vi "Fade.vi"(6 "Fade (Exponential)":T1, 8 "error in":errorcluster, 9 "Target Transparency (0)":u8, 10 "Fade time (ms)":variant, 11 "VI Reference (calling VI)":refnum<vi>) -> (0 "error out":errorcluster, 3 "dup VI Reference":refnum<vi>)   [LabVIEW 2012]
doc: "Produces a fade in or out, from the actual value to the target transparency. Use this generic VI when you start from an unknown transparency value.\n\nVariant (%) can be a numeric or a string containing a number. This allows the use of string-based arguments without the need to convert to a number."
uses:
  _fadetype.ctl
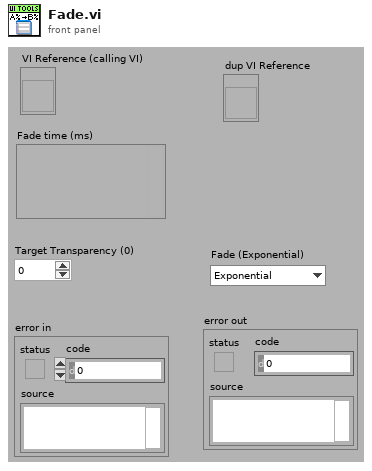
[diagram p1: front panel]
types:
  T1 = typedef "_fadetype.ctl" = enum16{"Exponential", "Linear"}
  T2 = typedef "Type Descriptor Enumeration__ogtk.ctl" = enum8{"<Null>", "I8", "I16", "I32", "I64", "U8", "U16", "U32", "U64", "SGL", "DBL", "EXT", "CSG", "CDB", "CXT", "0x0F", "0x10", "0x11", "0x12", "0x13", "0x14", "Enum U8", "Enum U16", "Enum U32", "Enum U64", "SGL PQ", "DBL PQ", "EXT PQ", "CSG PQ", "CDB PQ", "CXT PQ", "0x1F", "0x20", "Boolean", "0x22", "0x23", "0x24", "0x25", "0x26", "0x27", "0x28", "0x29", "0x2A", "0x2B", "0x2C", "0x2D", "0x2E", "0x2F", "String", "0x31", "Path", "Pict", "0x34", "0x35", "0x36", "DAQ", "0x38", "0x39", "0x3A", "0x3B", "0x3C", "0x3D", "0x3E", "0x3F", "Array", "0x41", "0x42", "0x43", "0x44", "0x45", "0x46", "0x47", "0x48", "0x49", "0x4A", "0x4B", "0x4C", "0x4D", "0x4E", "0x4F", "Cluster", "0x51", "0x52", "Variant", "Waveform", "0x55", "0x56", "0x57", "0x58", "0x59", "0x5A", "0x5B", "0x5C", "0x5D", "0x5E", "0x5F", "0x60", "0x61", "0x62", "0x63", "0x64", "0x65", "0x66", "0x67", "0x68", "0x69", "0x6A", "0x6B", "0x6C", "0x6D", "0x6E", "0x6F", "Refnum"}
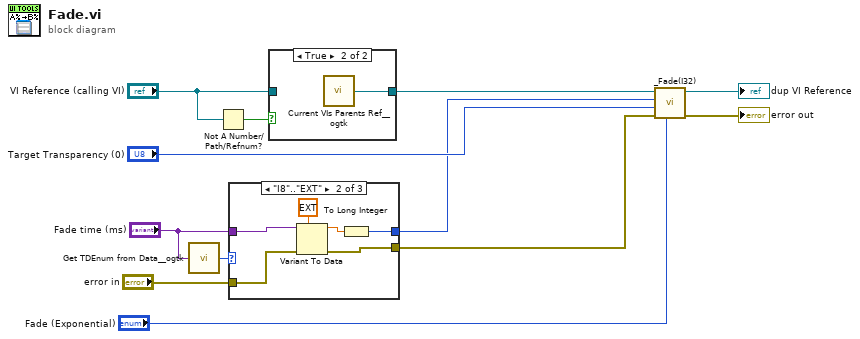
[diagram p0: block diagram]
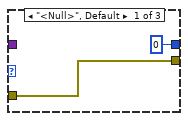
[diagram p3: hidden frame]
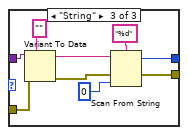
[diagram p4: hidden frame]
diagram:
  n1 = call <userlib>:"Get TDEnum from Data__ogtk.vi"("Data"="Fade time (ms)") -> ("Type Descriptor Enumeration"=w12:T2)  [unwired: 4 out]
  n2 = Not A Number/Path/Refnum?(number/path/refnum="VI Reference (calling VI)") -> (NaN/Path/Refnum?=w9:bool)
  n3 = case shown="\"I8\"..\"EXT\"" w12 {
    tunnel: "Fade time (ms)" -> [_ w20 w29]
    tunnel: [0 w17 w26] -> w1
    tunnel: [w13 w16 w21] -> w3
    tunnel: "error in" -> [w13 w15 w22]
    frame "<Null>", Default {
    }
    frame "I8".."EXT" {
      n4 = Variant To Data(error in=w15, type=ext 0.0 ("Front Panel Window:Transparency"), Variant=w20) -> (data=w18:ext, error out=w16:errorcluster)
      n5 = To Long Integer(number=w18) -> (32bit integer=w17:i32)
    }
    frame "String" {
      n6 = Variant To Data(error in=w22, type="" ("Front Panel Window:Transparency"), Variant=w29) -> (data=w23:string, error out=w24:errorcluster)
      n7 = Scan From String(format string="%d", input string=w23, error in=w24, default 1=0 ("Front Panel Window:Transparency")) -> (error out=w21:errorcluster, output 1=w26:i32)  [unwired: 1 in, 2 out]
    }
  }
  n8 = case shown="True" w9 {
    tunnel: "VI Reference (calling VI)" -> [w30 _]
    tunnel: [w30 w31] -> w4
    frame False {
    }
    frame True {
      n9 = call <userlib>:"Current VIs Parents Ref__ogtk.vi"() -> ("Calling VI's Reference"=w31:refnum<vi>)  [unwired: 2 out]
    }
  }
  n10 = call "_Fade(I32).vi"("Fade (Exponential)"="Fade (Exponential)", "error in"=w3, "Target Transparency (0)"="Target Transparency (0)", "Fade time (ms)"=w1, "VI Reference (calling VI)"=w4) -> ("error out"=→"error out":errorcluster, "dup VI Reference"=→"dup VI Reference":refnum<vi>)  [unwired: 5 out]
